vi "PM_Set-Get_Avg.vi"(8 "error in (no error)":errorcluster {"code" format="%.0x"}, 10 "Average counts":dbl caption="Average Time (0.0)") -> (0 "error out":errorcluster, 2 "Average counts":dbl caption="Average Time")   [LabVIEW 2018]
uses:
  Control 1.ctl
panel:
  out "Sensor Name":string
  out "Power":dbl
  in  "Wavelength":dbl caption="Wavelength (0.0)"
  out "Wavelength":dbl
  in  "instrument handle":refnum<visa-resource-name>
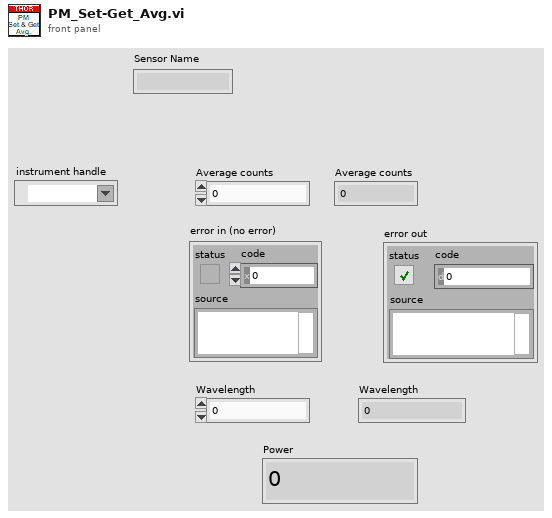
[diagram p1: front panel]
types:
  T1 = typedef "Control 1.ctl" = enum16{"Init", "Set-Get Average", "Set-Get Wavelength", "Do Measure", "Idle", "Uninit"}
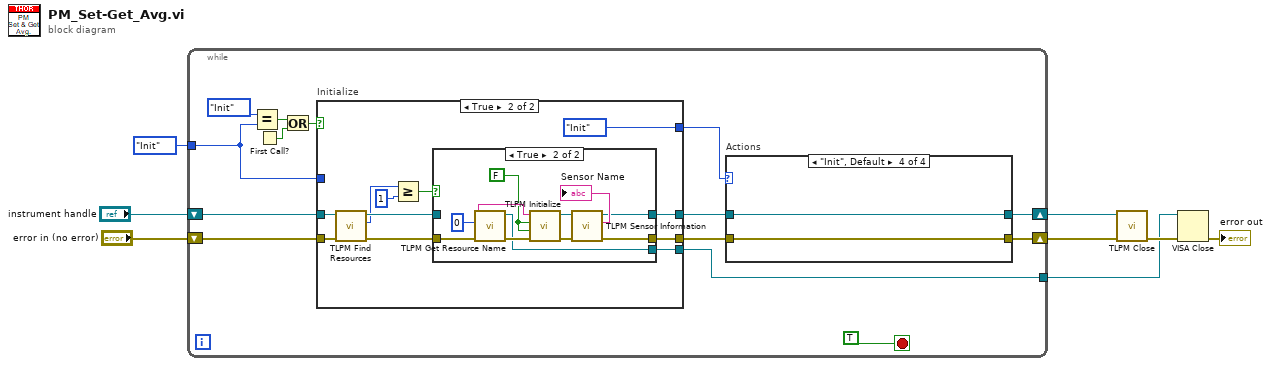
[diagram p0: block diagram]
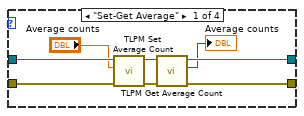
[diagram p2: hidden frame]
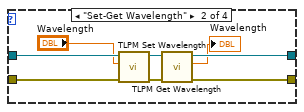
[diagram p3: hidden frame]
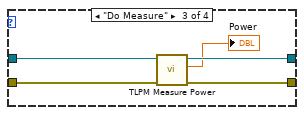
[diagram p4: hidden frame]
diagram:
  n1 = while {
    shift-right: [w12] -> w4
    shift-left: "error in (no error)" -> [w20]
    tunnel: Control_1."Init" -> [w15]
    shift-right: [w13] -> w1
    shift-left: "instrument handle" -> [w21]
    tunnel: [w10] -> w2
    stop <- TRUE stop-if-true
    n2 = Equal?(x=Control_1."Init" ("y"), y=w15) -> (x = y?=w19:bool)
    n3 = First Call?() -> (First Call?: T/F=w18:bool)
    n4 = Or(x=w19, y=w18) -> (x .or. y?=w17:bool)
    n5 = case "Initialize" shown="True" w17 {
      tunnel: w21 -> [w46 w58]
      tunnel: [w47 w56] -> w14
      tunnel: w20 -> [w47 w52]
      tunnel: w15 -> [_ _]
      tunnel: [w46 w57] -> w11
      tunnel: [_ w49] -> w10
      tunnel: [_ Control_1."Init" ("y")] -> w9
      frame False {
      }
      frame True {
        n6 = call "TLPM Find Resources.vi"("error in (no error)"=w52, "instrument handle"=w58) -> ("error out"=w51:errorcluster, "Resource Count"=w50:u32, "instrument handle out"=w53:refnum<visa-resource-name>)  [unwired: 7 in]
        n7 = Greater Or Equal?(x=w50, y=u32 1) -> (x >= y?=w54:bool)
        n8 = case shown="True" w54 {
          tunnel: w51 -> [w59 w71]
          tunnel: w53 -> [w60 _]
          tunnel: [w60 w63] -> w57
          tunnel: [w59 w62] -> w56
          tunnel: [_ w61] -> w49
          frame False {
          }
          frame True {
            w68 = FALSE ("ID Query (Do Query)")
            n9 = call "TLPM Get Resource Name.vi"("error in (no error)"=w71, "Index (0)"=u32 0) -> ("error out"=w70:errorcluster, "instrument handle out"=w61:refnum<visa-resource-name>, "Resource Name"=w69:string)  [unwired: 7 in]
            n10 = call "TLPM Initialize.vi"("error in (no error)"=w70, "Reset Device (Reset Device)"=w68, "ID Query (Do Query)"=w68, "resource name"=w69) -> ("error out"=w66:errorcluster, "instrument handle out"=w65:refnum<visa-resource-name>)  [unwired: 6 in]
            n11 = call "TLPM Sensor Information.vi"("error in (no error)"=w66, "instrument handle"=w65) -> ("error out"=w62:errorcluster, "Sensor Name"=→"Sensor Name":string, "instrument handle out"=w63:refnum<visa-resource-name>)  [unwired: 2 in, 5 out]
          }
        }
      }
    }
    n12 = case "Actions" shown="\"Init\", Default" w9 {
      tunnel: w11 -> [w30 w38 w43 w44]
      tunnel: w14 -> [w29 w33 w40 w45]
      tunnel: [w25 w36 w42 w44] -> w13
      tunnel: [w26 w31 w39 w45] -> w12
      frame "Set-Get Average" {
        n13 = call "TLPM Set Average Count.vi"("error in (no error)"=w29, "Average Count (1)"="Average counts", "instrument handle"=w30) -> ("error out"=w27:errorcluster, "instrument handle out"=w28:refnum<visa-resource-name>)  [unwired: 7 in]
        n14 = call "TLPM Get Average Count.vi"("error in (no error)"=w27, "instrument handle"=w28) -> ("error out"=w26:errorcluster, "Average Count"=→"Average counts":i16, "instrument handle out"=w25:refnum<visa-resource-name>)  [unwired: 7 in]
      }
      frame "Set-Get Wavelength" {
        n15 = call "TLPM Set Wavelength.vi"("error in (no error)"=w33, "Wavelength (0.0)"="Wavelength", "instrument handle"=w38) -> ("error out"=w32:errorcluster, "instrument handle out"=w37:refnum<visa-resource-name>)  [unwired: 7 in]
        n16 = call "TLPM Get Wavelength.vi"("error in (no error)"=w32, "instrument handle"=w37) -> ("error out"=w31:errorcluster, "Wavelength"=→"Wavelength":dbl, "instrument handle out"=w36:refnum<visa-resource-name>)  [unwired: 7 in]
      }
      frame "Do Measure" {
        n17 = call "TLPM Measure Power.vi"("error in (no error)"=w40, "instrument handle"=w43) -> ("error out"=w39:errorcluster, "Power"=→"Power":dbl, "instrument handle out"=w42:refnum<visa-resource-name>)  [unwired: 7 in]
      }
      frame "Init", Default {
      }
    }
  }
  n18 = call "TLPM Close.vi"("error in (no error)"=w4, "instrument handle"=w1) -> ("error out"=w3:errorcluster)  [unwired: 9 in]
  n19 = VISA Close(VISA resource name=w2, error in (no error)=w3) -> (error out=→"error out":errorcluster)
